vi "PCO_Grab_v2.vi"() -> ()   [LabVIEW 2026]
doc: "This example demonstrates the image acquisition with one camera in ring buffer mode together with a live display of the latest images during record. After record is stopped, the images can be addressed by index.\nNote that this example will not be fail save, i.e. doesnt react on errors, just handles them forward to the end\n\nUsage:\nSelect your required image count, data format and the camera setup before you start the program.\nOnce started, the camera class will be initialized and images will be recorded and displayed automatically\nYou can stop the images by pressing stop record.\nAfter stopped, the image at the selected index will be read out\nTo finish the program click on quit application, this will force an exit of the camera class\nYou can change your required ROI after and also during the record."
uses:
  <instrlib>/PCO_SDK/File Group 0/vi.lib/Excelitas PCO GmbH/pco.labview/camera/Camera.lvclass
  <instrlib>/PCO_SDK/File Group 0/vi.lib/Excelitas PCO GmbH/pco.labview/pco.sdk/TimingControl/TimingControl.lvlib
panel:
  out "x = y ?":bool
  out "Image":picture
  out "Image(U16)":u16[][](graph)
  in  "data_format":T1(ring)=enum."Mono16"
  in  "Image Index":u32 max=110 step=1
  out "Recorded Images":u32=1
  in  "Quit":bool
  out "Error":errorcluster={"status"=FALSE, "code"=0, "source"="OK."} {"code" format="%x"}
  in  "roiY1":u64=2048 min=1 max=2048 step=1
  in  "roiX1":u64=2048 min=1 max=2048 step=1
  in  "roiY0":u64=1 min=1 max=2047 step=1
  in  "roiX0":u64=1 min=1 max=2047 step=1
  in  "dwImgCount":u32=10 caption="Required Number of Images" max=2397
  # "This example demonstrates the image acquisition with one camera in ring buffer mode together with a live display of the latest images during record. After record is stopped, the images can be addressed by index.\nNote that this example will not be fail save, i.e. doesnt react on errors, just handles them forward to the end\n\nUsage:\nSelect your required image count, data format and the camera setup before you start the program.\nOnce started, the camera class will be initialized and images will be recorded and displayed automatically\nYou can stop the images by pressing stop record.\nAfter stopped, the image at the selected index will be read out\nTo finish the program click on quit application, this will force an exit of the camera class\nYou can change your required ROI after and also during the record."
  # "pco.labview"
  # "Camera Setup"
  # "Recording Control"
  # "Parameters for image readout"
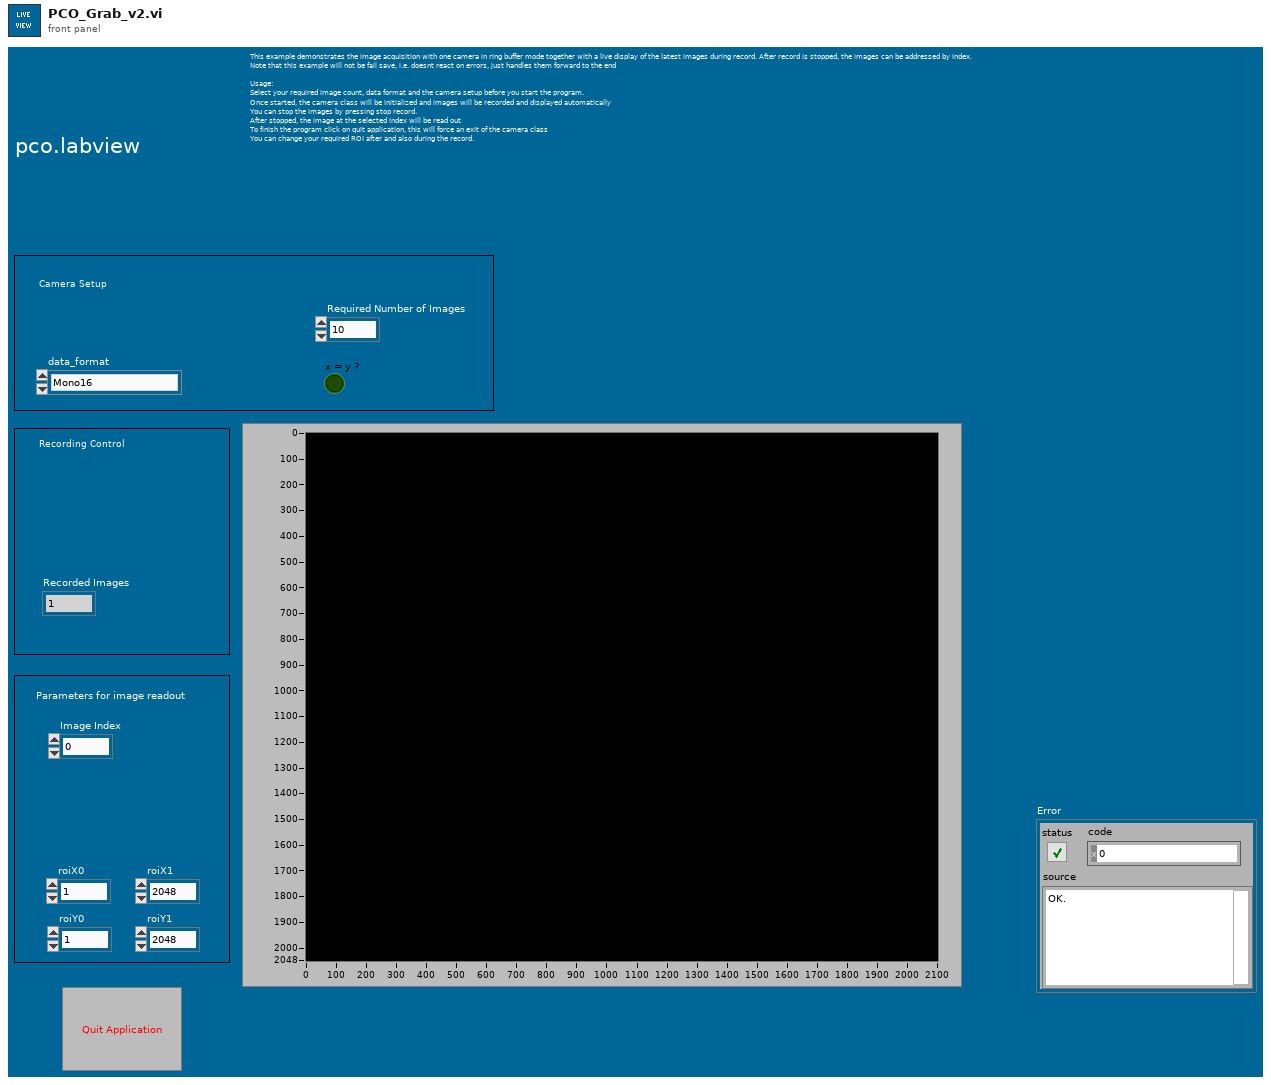
[diagram p1: front panel]
types:
  T1 = enum16{"Undefined", "Mono8", "Mono16", "BGRA8", "RGBA8", "BGRA16", "RGBA16", "CompressedMono8"}
  T2 = enum16{"sequence", "sequence non blocking", "ring buffer", "fifo", "sequence_dpcore", "sequence_non_blocking_dpcore", "ring_buffer_dpcore", "fifo_dpcore", "tif", "multitif", "pcoraw", "b16", "dicom", "multidicom", "camram_ring", "camram_segment"}
  T3 = enum16{"auto sequence", "software trigger", "external exposure start", "external exposure control"}
  T4 = cluster{"wSignalNum":u16, "wEnabled":u16, "wType":u16, "wPolarity":u16, "wFilterSetting":u16, "wSelected":u16, "dwParameter":u32[], "dwSignalFunctionality":u32[]}
  T5 = typedef "Camera.lvclass/binning.ctl" = cluster{"vert":u16, "horz":u16, "mode":u16}
  T6 = cluster{"exposure_time_s":dbl, "delay_time_s":dbl, "roi":cluster{"x0":u64, "y0":u64, "x1":u64, "y1":u64}, "timestamp_mode":u16, "pixelrate":u32, "trigger_mode":u16, "acquire_mode":u16, "metadata_mode":u16, "noisefilter_mode":u16, "pixel_format":u32, "binning":T5, "auto_exposure":cluster{"region":u16, "min_exposure_s":dbl, "max_exposure_s":dbl}}
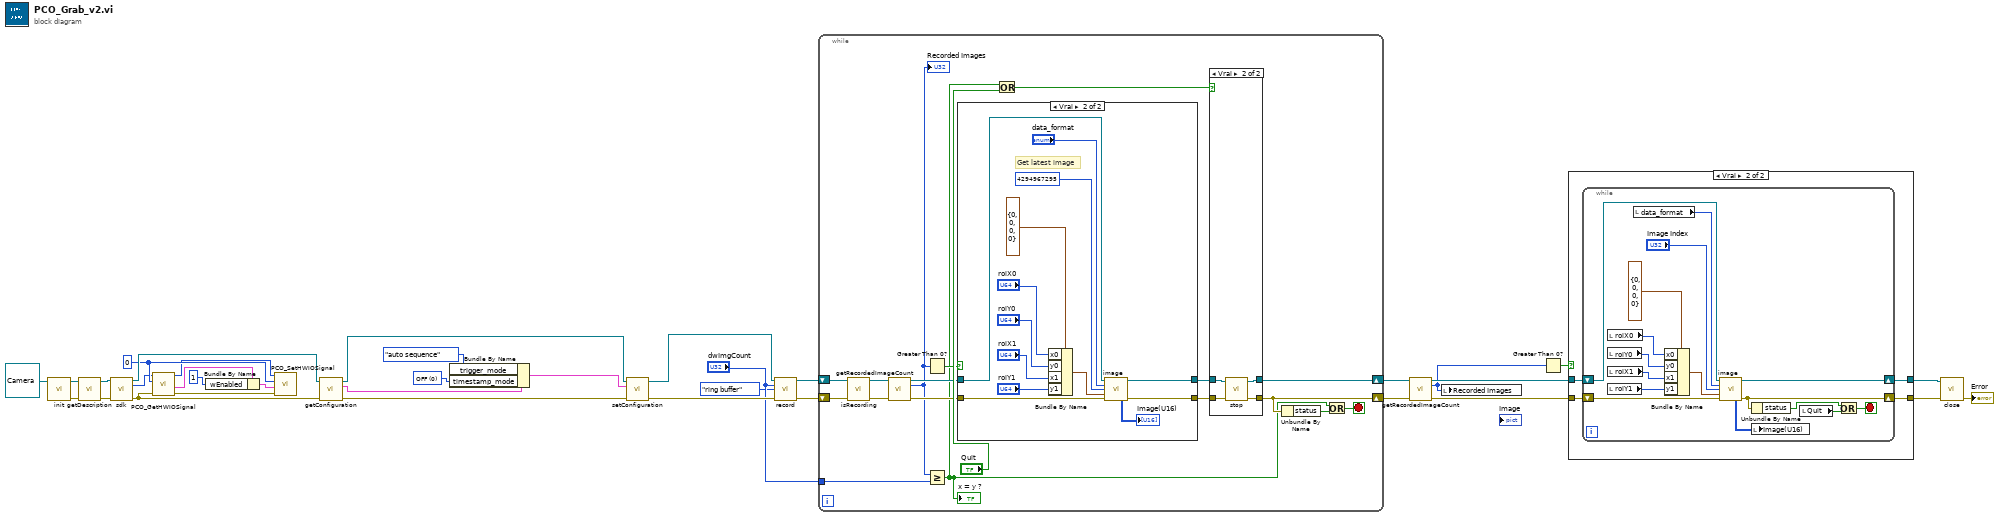
[diagram p0: block diagram]
diagram:
  w8 = u16 0 items=["OFF", "Binary", "Binary+ASCII", "ASCII"] ("wTimeStampMode")
  w14 = u16 0 ("wSignalNum")
  n1 = call-dynamic "init.vi"("Camera in"=refnum<class "Camera.lvclass"> refnum) -> ("Camera out"=w19:refnum<class "Camera.lvclass">, "error out"=w20:errorcluster)  [unwired: 8 in]
  n2 = call-dynamic "getDescription.vi"("error in (no error)"=w20, "Camera in"=w19) -> ("error out"=w18:errorcluster, "Camera out"=w17:refnum<class "Camera.lvclass">)  [unwired: 7 in, 1 out]
  n3 = call-dynamic "sdk.vi"("Camera in"=w17, "error in (no error)"=w18) -> ("Camera out"=w30:refnum<class "Camera.lvclass">, "sdk"=w10:u64, "error out"=w29:errorcluster)  [unwired: 11 in]
  n4 = call <instrlib>:"PCO_GetHWIOSignal.vi"("error in (no error)"=w29, "wSignalNum"=w14, "ph"=w10) -> ("error out"=w12:errorcluster, "strSignal"=w16:T4, "ph out"=w11:u64)  [unwired: 5 in, 1 out]
  n5 = Bundle By Name(cluster=w16, "wEnabled"=u16 1) -> (w13:T4)
  n6 = call <instrlib>:"PCO_SetHWIOSignal.vi"("error in (no error)"=w12, "strSignal"=w13, "wSignalNum"=w14, "ph"=w11) -> ()  [unwired: 5 in, 3 out]
  n7 = call-dynamic "getConfiguration.vi"("error in (no error)"=w29, "Camera in"=w30) -> ("error out"=w4:errorcluster, "configuration"=w9:T6, "Camera out"=w6:refnum<class "Camera.lvclass">)  [unwired: 7 in]
  n8 = Bundle By Name(cluster=w9, "trigger_mode"=T3."auto sequence" ("TriggerMode"), "timestamp_mode"=w8) -> (w5:T6)
  n9 = call-dynamic "setConfiguration.vi"("error in (no error)"=w4, "configuration"=w5, "Camera in"=w6) -> ("error out"=w34:errorcluster, "Camera out"=w35:refnum<class "Camera.lvclass">)  [unwired: 7 in]
  n10 = call-dynamic "record.vi"("Camera in"=w35, "num_images"="dwImgCount", "record_mode"=T2."ring buffer", "error in (no error)"=w34) -> ("Camera out"=w23:refnum<class "Camera.lvclass">, "error out"=w22:errorcluster)  [unwired: 10 in]
  n11 = while {
    shift-right: [w40] -> w33
    shift-left: w22 -> [w42]
    shift-right: [w41] -> w28
    shift-left: w23 -> [w43]
    tunnel: "dwImgCount" -> [w37]
    stop <- w51 stop-if-true
    n12 = call-dynamic "isRecording.vi"("Camera in"=w43, "error in (no error)"=w42) -> ("Camera out"=w48:refnum<class "Camera.lvclass">, "error out"=w47:errorcluster)  [unwired: 11 in, 1 out]
    n13 = call-dynamic "getRecordedImageCount.vi"("Camera in"=w48, "error in (no error)"=w47) -> ("Camera out"=w45:refnum<class "Camera.lvclass">, "recorded_image_count"=w38:u32, "error out"=w46:errorcluster)  [unwired: 11 in]
    "Recorded Images" <- w38
    n14 = Greater Than 0?(x=w38) -> (x > 0?=w39:bool)
    n15 = Greater Or Equal?(x=w38, y=w37) -> (x >= y?=w36:bool)
    "x = y ?" <- w36
    n16 = case shown="Vrai" w39 {
      tunnel: [w54 w63] -> w49
      tunnel: w46 -> [w54 w60]
      tunnel: w45 -> [w55 w59]
      tunnel: [w55 w58] -> w44
      frame False {
      }
      frame True {
        # "Get latest image"
        n17 = Bundle By Name(cluster=cluster{"x0":u64, "y0":u64, "x1":u64, "y1":u64} {"x0"=0, "y0"=0, "x1"=0, "y1"=0} ("roi"), "x0"="roiX0", "y0"="roiY0", "x1"="roiX1", "y1"="roiY1") -> (w64:cluster{"x0":u64, "y0":u64, "x1":u64, "y1":u64})
        n18 = call-dynamic "image.vi"("Camera in"=w59, "data_format"="data_format", "image_index"=u32 4294967295 ("dwImgIdx"), "roi"=w64, "error in (no error)"=w60) -> ("Camera out"=w58:refnum<class "Camera.lvclass">, "raw_image (U16)"=→"Image(U16)":u16[][], "error out"=w63:errorcluster)  [unwired: 2 in, 6 out]
      }
    }
    n19 = Or(x=w36, y="Quit") -> (x .or. y?=w52:bool)
    n20 = case shown="Vrai" w52 {
      tunnel: w49 -> [w70 w71]
      tunnel: [w69 w73] -> w41
      tunnel: [w70 w74] -> w40
      tunnel: w44 -> [w69 w72]
      frame False {
      }
      frame True {
        n21 = call-dynamic "stop.vi"("error in (no error)"=w71, "Camera in"=w72) -> ("error out"=w74:errorcluster, "Camera out"=w73:refnum<class "Camera.lvclass">)  [unwired: 8 in]
      }
    }
    n22 = Unbundle By Name(w40) -> ("status"=w50:bool)
    n23 = Or(x=w36, y=w50) -> (x .or. y?=w51:bool)
  }
  n24 = call-dynamic "getRecordedImageCount.vi"("Camera in"=w28, "error in (no error)"=w33) -> ("Camera out"=w27:refnum<class "Camera.lvclass">, "recorded_image_count"=w25:u32, "error out"=w32:errorcluster)  [unwired: 11 in]
  n25 = local write "Recorded Images"(w25) -> ()
  n26 = Greater Than 0?(x=w25) -> (x > 0?=w2:bool)
  n27 = case shown="Vrai" w2 {
    tunnel: w32 -> [w75 w80]
    tunnel: [w75 w79] -> w31
    tunnel: w27 -> [w76 w78]
    tunnel: [w76 w77] -> w26
    frame False {
    }
    frame True {
      n28 = while {
        shift-right: [w88] -> w79
        shift-left: w80 -> [w96]
        shift-right: [w82] -> w77
        shift-left: w78 -> [w83]
        stop <- w90 stop-if-true
        n29 = local read "roiX0"() -> (w86:u64)
        n30 = local read "roiY0"() -> (w87:u64)
        n31 = local read "roiX1"() -> (w94:u64)
        n32 = local read "roiY1"() -> (w93:u64)
        n33 = local read "data_format"() -> (w84:T1)
        n34 = Bundle By Name(cluster=cluster{"x0":u64, "y0":u64, "x1":u64, "y1":u64} {"x0"=0, "y0"=0, "x1"=0, "y1"=0} ("roi"), "x0"=w86, "y0"=w87, "x1"=w94, "y1"=w93) -> (w95:cluster{"x0":u64, "y0":u64, "x1":u64, "y1":u64})
        n35 = call-dynamic "image.vi"("Camera in"=w83, "data_format"=w84, "image_index"="Image Index", "roi"=w95, "error in (no error)"=w96) -> ("Camera out"=w82:refnum<class "Camera.lvclass">, "raw_image (U16)"=w81:u16[][], "error out"=w88:errorcluster)  [unwired: 2 in, 6 out]
        n36 = Unbundle By Name(w88) -> ("status"=w91:bool)
        n37 = local write "Image(U16)"(w81) -> ()
        n38 = local read "Quit"() -> (w92:bool)
        n39 = Or(x=w91, y=w92) -> (x .or. y?=w90:bool)
      }
    }
  }
  n40 = call-dynamic "close.vi"("error in (no error)"=w31, "Camera in"=w26) -> ("error out"=→"Error":errorcluster)  [unwired: 9 in]
